vi "ModifyImage ctab.vi"(4 "maximum":dbl, 6 "minimum":dbl, 8 "error in (no error)":errorcluster, 9 "Invert Color Scheme? [NO]":bool, 10 "Color Table Name [Rainbow]":string="Rainbow", 11 "ITX Commands in":refnum<class "ITX Commands.lvclass">) -> (0 "error out":errorcluster, 3 "ITX Commands out":refnum<class "ITX Commands.lvclass">)   [LabVIEW 2019, in "ITX Commands.lvclass"]
uses:
  ITX Commands.lvclass
panel:
  out "resulting string":string="ModifyImage '' ctab{,, Rainbow, 0}"
  # "Some Example Color Table Names \n(More on pg. 401 of Igor manual):"
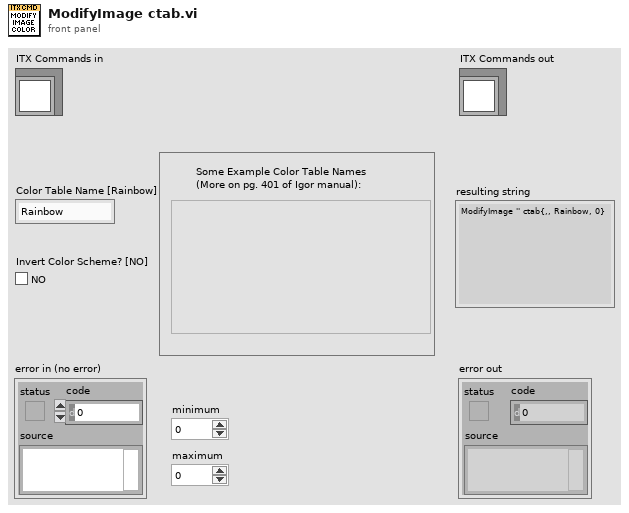
[diagram p1: front panel]
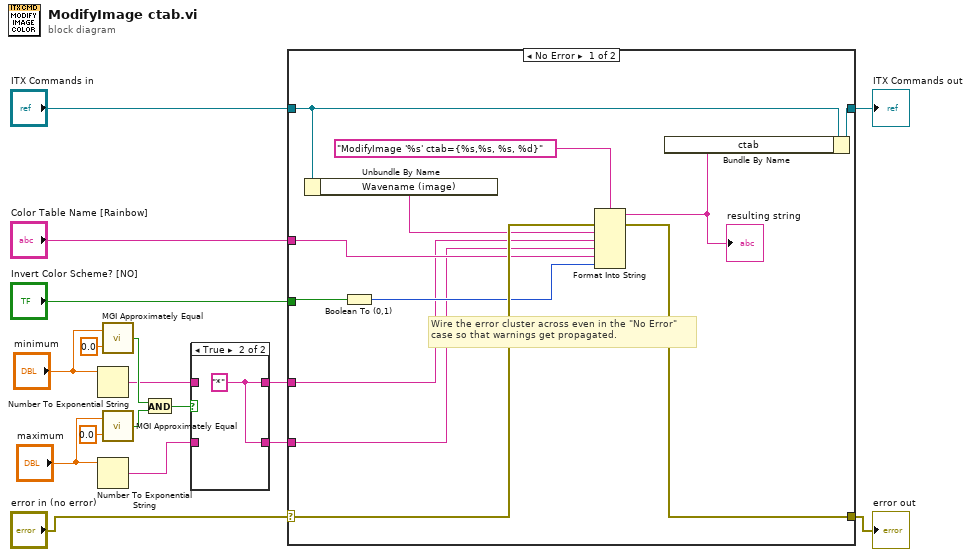
[diagram p0: block diagram]
diagram:
  n1 = Number To Exponential String(number="minimum") -> (E-format string=w2:string)  [unwired: 3 in]
  n2 = Number To Exponential String(number="maximum") -> (E-format string=w3:string)  [unwired: 3 in]
  n3 = call "MGI Approximately Equal.vi"("Numeric 2"=0.0, "Numeric 1"="minimum") -> ("approx = ?"=w6:bool)
  n4 = call "MGI Approximately Equal.vi"("Numeric 2"=0.0, "Numeric 1"="maximum") -> ("approx = ?"=w7:bool)
  n5 = And(x=w6, y=w7) -> (x .and. y?=w1:bool)
  n6 = case shown="True" w1 {
    tunnel: [w19 w20] -> w5
    tunnel: [w18 w20] -> w4
    tunnel: w3 -> [w18 _]
    tunnel: w2 -> [w19 _]
    frame False {
    }
    frame True {
      w20 = "*" ("t")
    }
  }
  n7 = case shown="No Error" "error in (no error)" {
    selector: "error in (no error)" -> [w27 w34]
    tunnel: [w26 w34] -> w16
    tunnel: [w28 w33] -> w14
    tunnel: "ITX Commands in" -> [w29 w33]
    tunnel: "Color Table Name [Rainbow]" -> [w23 _]
    tunnel: "Invert Color Scheme? [NO]" -> [w31 _]
    tunnel: w5 -> [w22 _]
    tunnel: w4 -> [w21 _]
    frame No Error {
      # "Wire the error cluster across even in the \"No Error\"\ncase so that warnings get propagated."
      n8 = Unbundle By Name(w29) -> ("Wavename (image)"=w25:string)
      n9 = Boolean To (0,1)(Boolean=w31) -> (0, 1=w24:i16)
      n10 = Format Into String(format string="ModifyImage '%s' ctab={%s,%s, %s, %d}", error in=w27, w25, w22, w21, w23, w24) -> (resulting string=w30:string, error out=w26:errorcluster)  [unwired: 1 in]
      "resulting string" <- w30
      n11 = Bundle By Name(cluster=w29, "ctab"=w30) -> (w28:refnum<class "ITX Commands.lvclass">)
    }
    frame Error {
    }
  }
  "error out" <- w16
  "ITX Commands out" <- w14
